vi "connect_subscribe.vi"(8 "错误输入（无错误）":errorcluster, 9 "type":string="std_msgs/String", 10 "topic":string="/chatter", 11 "address":string="192.168.1.134") -> (0 "错误输出":errorcluster, 3 "连接ID输出":refnum<k5>)   [LabVIEW 2014]
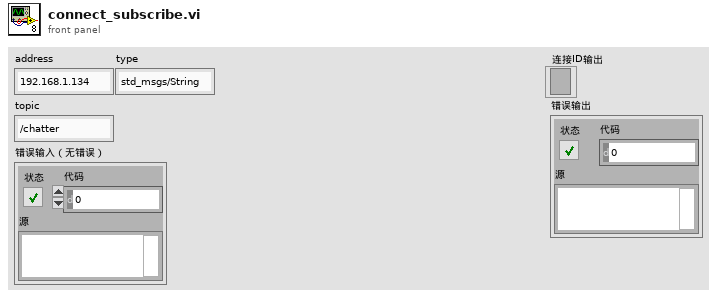
[diagram p1: front panel]
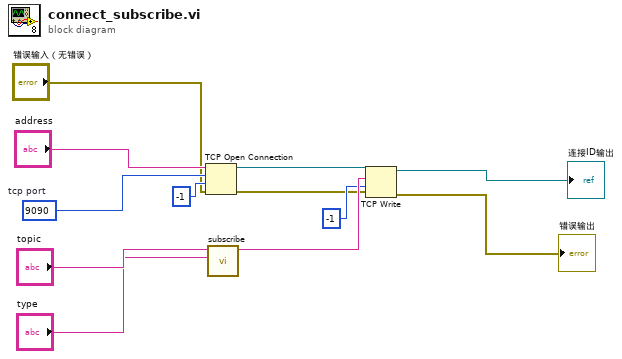
[diagram p0: block diagram]
diagram:
  w12 = u16 9090  # tcp port
  n1 = TCP Open Connection(address="address", remote port or service name=w12, timeout ms (60000)=-1 ("超时毫秒(60000)"), error in (no error)="错误输入（无错误）") -> (connection ID=w7:refnum<k5>, error out=w2:errorcluster)  [unwired: 1 in]
  n2 = call "subscribe.vi"("type"="type", "topic"="topic") -> ("JSON字符串"=w6:string)  [unwired: 9 in]
  n3 = TCP Write(connection ID=w7, data in=w6, error in (no error)=w2, 9:-1 ("超时毫秒(25000)")) -> (connection ID out=→"连接ID输出":refnum<k5>, error out=→"错误输出":errorcluster)  [unwired: 1 out]
